vi "Grava_EQ_report_u.vi"(1 "EQ Data+Report_u (hex)":u32[](array[numeric]) format="%x", 2 "ChipID (file name)":string, 3 "EQ_u folder path":path) -> ()   [LabVIEW 2015, in "VIPM2.lvlib"]
doc: "Partint del array hex EQ DATA+REPORT d'<b>un sol chip</b>, passa els valors numerics hex a integer i els grava en un archiu ChipID_report.txt; per a fàcil lectura per l'usuari.\nInclou el report de pixels bons."
uses:
  VIPM2.lvlib
panel:
  out "EQ Report (hex)":u32[](array[numeric])
  out "EQ Report integer":string[][](array[string])
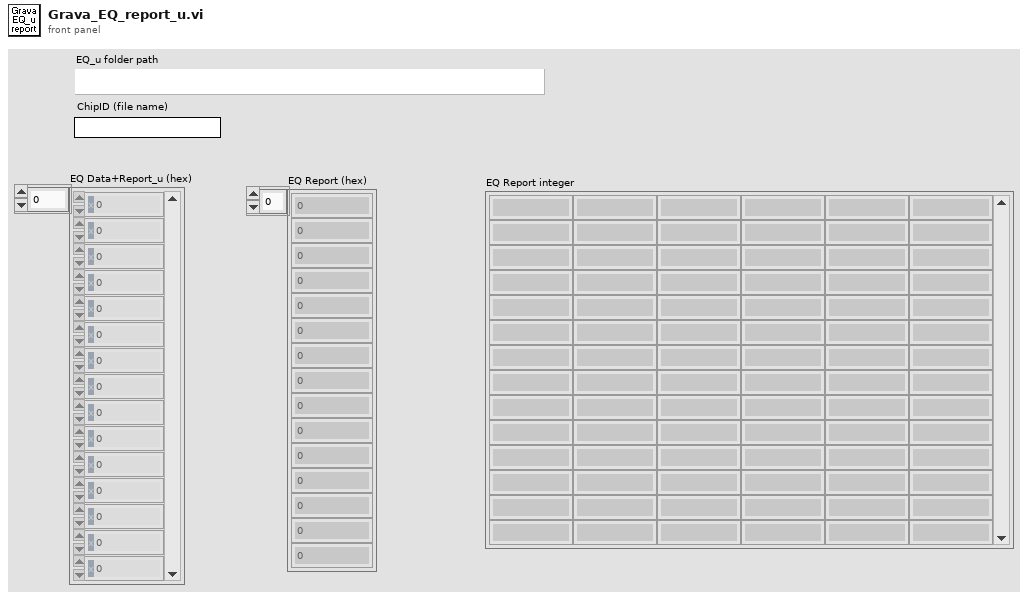
[diagram p1: front panel]
types:
  T1 = enum16{"open", "replace", "create", "open or create", "replace or create", "replace or create with confirmation"}
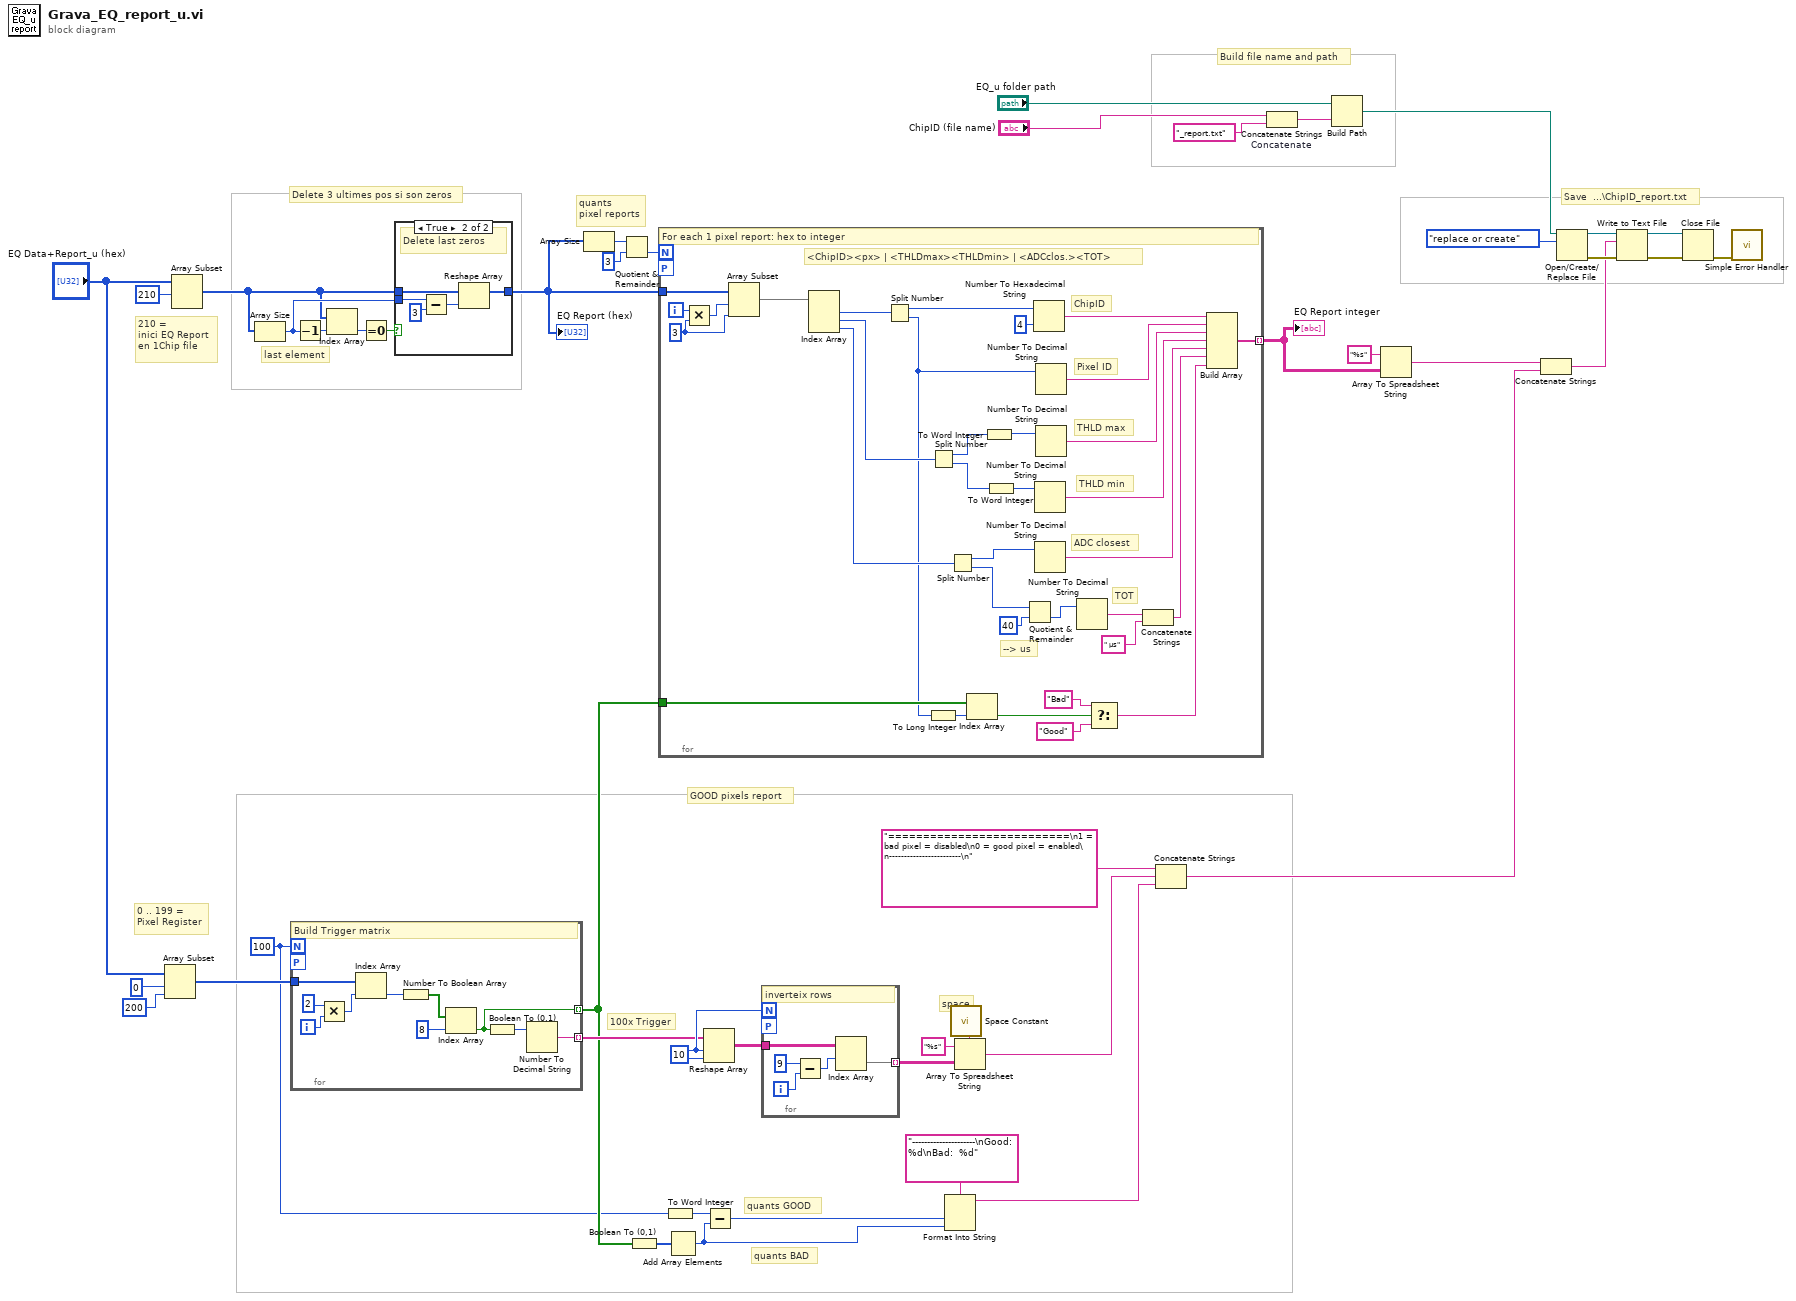
[diagram p0: block diagram]
diagram:
  w21 = 10 ("dimension size")
  w9 = 100
  # "quants GOOD"
  # "quants BAD"
  # "GOOD pixels report"
  # "100x Trigger"
  # "0 .. 199 =\nPixel Register"
  # "space"
  # "Delete 3 ultimes pos si son zeros"
  # "last element"
  # "Save  ...\\ChipID_report.txt"
  # "Build file name and path"
  # "quants\npixel reports"
  # "210 = \ninici EQ Report\nen 1Chip file"
  n1 = Array Subset "Array Subset"(array="EQ Data+Report_u (hex)", index=0, length=200) -> (w14:u32[])
  n2 = Array Subset "Array Subset"(array="EQ Data+Report_u (hex)", index=210 ("offset (0)")) -> (w28:u32[])  [unwired: 1 in]
  n3 = Array Size(array=w28) -> (size(s)=w32:i32)
  n4 = for {
    N: w9 -> [_]
    tunnel: w14 -> [w56]
    tunnel: [w49] -> w13 mode=indexing
    tunnel: [w47] -> w12 mode=indexing
    workers-P: _ -> [_]
    i -> [w52]
    # "Build Trigger matrix"
    n5 = Multiply(x=2 ("y"), y=w52) -> (x*y=w55:i32)
    n6 = Index Array "Index Array"(array=w56, index=w55) -> (element=w54:u32)
    n7 = Number To Boolean Array(number=w54) -> (Boolean array=w51:bool[])
    n8 = Index Array "Index Array"(array=w51, index=8) -> (element=w47:bool)
    n9 = Boolean To (0,1)(Boolean=w47) -> (0, 1=w48:i16)
    n10 = Number To Decimal String(number=w48) -> (decimal integer string=w49:string)  [unwired: 1 in]
  }
  n11 = Decrement(x=w32) -> (x-1=w30:i32)
  n12 = Index Array(array=w28, index=w30) -> (element=w31:u32)
  n13 = Equal To 0?(x=w31) -> (x = 0?=w33:bool)
  n14 = case shown="True" w33 {
    tunnel: w28 -> [w57 w62]
    tunnel: [w57 w61] -> w29
    tunnel: w32 -> [_ w59]
    frame False {
    }
    frame True {
      # "Delete last zeros"
      n15 = Subtract(x=w59, y=3 ("length")) -> (x-y=w58:i32)
      n16 = Reshape Array "Reshape Array"(w62, w58) -> (w61:u32[])
    }
  }
  "EQ Report (hex)" <- w29
  n17 = Array Size(array=w29) -> (size(s)=w34:i32)
  n18 = Quotient & Remainder(x=w34, y=3) -> (floor(x/y)=w45:i32)  [unwired: 1 out]
  n19 = Boolean To (0,1)(Boolean=w12) -> (0, 1=w11:i16[])
  n20 = for {
    N: w45 -> [_]
    tunnel: w29 -> [w84]
    tunnel: [w91] -> w44 mode=indexing
    tunnel: w12 -> [w73]
    workers-P: _ -> [_]
    i -> [w96]
    w83 = 3 ("y")
    # "--> us"
    # "<ChipID><px> | <THLDmax><THLDmin> | <ADCclos.><TOT>"
    # "TOT"
    # "ADC closest"
    # "THLD min"
    # "THLD max"
    # "Pixel ID"
    # "ChipID"
    # "For each 1 pixel report: hex to integer"
    n21 = Multiply(x=w96, y=w83) -> (x*y=w85:i32)
    n22 = Array Subset "Array Subset"(array=w84, index=w85, length=w83) -> (w82:u32[])
    n23 = Index Array "Index Array"(array=w82) -> (element #1=w79:u32, element #2=w77:u32, element #3=w76:u32)  [unwired: 3 in]
    n24 = Split Number(x=w79) -> (hi(x)=w78:u16, lo(x)=w71:u16)
    n25 = To Long Integer(number=w71) -> (32bit integer=w72:i32)
    n26 = Split Number(x=w77) -> (hi(x)=w65:u16, lo(x)=w63:u16)
    n27 = Split Number(x=w76) -> (hi(x)=w75:u16, lo(x)=w74:u16)
    n28 = Index Array "Index Array"(array=w73, index=w72) -> (element=w70:bool)
    n29 = To Word Integer(number=w65) -> (16bit integer=w66:i16)
    n30 = To Word Integer(number=w63) -> (16bit integer=w64:i16)
    n31 = Quotient & Remainder(x=w74, y=u16 40) -> (floor(x/y)=w89:u16)  [unwired: 1 out]
    n32 = Number To Hexadecimal String(1:i16 4 ("width (-)"), 2:w78) -> (0:w80:string)
    n33 = Number To Decimal String(number=w64) -> (decimal integer string=w94:string)  [unwired: 1 in]
    n34 = Number To Decimal String(number=w75) -> (decimal integer string=w95:string)  [unwired: 1 in]
    n35 = Number To Decimal String(number=w71) -> (decimal integer string=w92:string)  [unwired: 1 in]
    n36 = Number To Decimal String(number=w66) -> (decimal integer string=w93:string)  [unwired: 1 in]
    n37 = Number To Decimal String(number=w89) -> (decimal integer string=w88:string)  [unwired: 1 in]
    n38 = Select(t="Bad", s=w70, f="Good") -> (s? t:f=w67:string)
    n39 = Concatenate Strings(w88, " µs" ("string")) -> (w86:string)
    n40 = Build Array(w80, w92, w93, w94, w95, w86, w67) -> (w91:string[])
  }
  "EQ Report integer" <- w44
  n41 = To Word Integer(number=w9) -> (16bit integer=w10:i16)
  n42 = Add Array Elements(numeric array=w11) -> (sum=w6:i16)
  n43 = Reshape Array "Reshape Array"(w13, w21, w21) -> (w22:string[][])
  n44 = Subtract(x=w10, y=w6) -> (x-y=w7:i16)
  n45 = for {
    N: w21 -> [_]
    tunnel: w22 -> [w101]
    tunnel: [w97] -> w20 mode=indexing
    workers-P: _ -> [_]
    i -> [w100]
    # "inverteix rows"
    n46 = Subtract(x=9, y=w100) -> (x-y=w98:i32)
    n47 = Index Array "Index Array"(array=w101, index (row)=w98) -> (element=w97:string[])  [unwired: 1 in]
  }
  n48 = Format Into String(format string="---------------------\nGood: %d\nBad:  %d", w7, w6) -> (resulting string=w5:string)  [unwired: 2 in, 1 out]
  n49 = call <vilib>:"Space Constant.vi"() -> ("String"=w18:string)
  n50 = Array To Spreadsheet String(delimiter (Tab)=w18, array=w20, 3:"%s" ("format string")) -> (spreadsheet string=w17:string)
  n51 = Concatenate Strings "Concatenate Strings"("==========================\n1 = bad pixel = disabled\n0 = good pixel = enabled\n------------------------\n", w17, w5) -> (w2:string)
  n52 = Concatenate Strings "Concatenate"("ChipID (file name)", "_report.txt" ("substring (\"\")")) -> (w26:string)
  n53 = Build Path(base path="EQ_u folder path", name or relative path=w26) -> (appended path=w36:path)
  n54 = Array To Spreadsheet String(array=w44, 3:"%s" ("format string")) -> (spreadsheet string=w4:string)  [unwired: 1 in]
  n55 = Concatenate Strings "Concatenate Strings"(w4, w2) -> (w3:string)
  n56 = Open/Create/Replace File(file path (use dialog)=w36, operation (0:open)=T1."replace or create") -> (refnum out=w41:refnum<file>, error out=w40:errorcluster)  [unwired: 4 in, 1 out]
  n57 = Write to Text File(file (use dialog)=w41, text=w3, error in=w40) -> (refnum out=w38:refnum<file>, error out=w39:errorcluster)  [unwired: 1 in, 1 out]
  n58 = Close File(refnum=w38, error in=w39) -> (error out=w37:errorcluster)  [unwired: 1 out]
  n59 = call <vilib>:"Simple Error Handler.vi"("error in (no error)"=w37) -> ()  [unwired: 4 in, 5 out]
